vi "Start Transfer.vi"(8 "error in (no error)":errorcluster, 9 "finite?":bool=TRUE, 10 "stream index":i32, 11 "refnum in":refnum<k20>) -> (0 "error out":errorcluster, 3 "refnum out":refnum<k20>)   [LabVIEW 2015, in "niInstr Streaming v1 Host.lvlib"]
doc: "This low-level VI directly pokes the state machine to a started state (defined by the <b>finite?</b> paramter. This VI still waits for the state machine to report that it has left the idle state to ensure that the transfer has actually been started by the FPGA.\n\nThis VI provides no error checking. It does not check the state prior to execution, which may result in undesired behavior if the FPGA is in a bad state to start with. This VI should only be used by clients when they are asserting that the configuration and state are valid prior to calling this VI. However, because no error checking is performed, this VI may improve performance for starting a transfer.\n\n<B>Input Parameters</B>\n\n<B>error in (no error)</B> 'error in' can accept error information wired from VIs previously called. Use this information to decide if any functionality should be bypassed in the event of errors from other VIs.\n\nRight-click the 'error in' control on the front panel and select 'Explain Error' or 'Explain Warning' from the shortcut menu for more information about the error.\n\n<B>finite?</B> Indicates that this transfer should use the previously configured number of samples to transfer.\n\n<B>stream index</B> Selects which stream index this VI will interface to. This is the index number at the end of the host interface controls (0..7).\n\n<B>Output Parameters</B>\n\n<B>error out</B> contains error information. This output provides standard error out functionality.\n\n<B>refnum out</B> Copy of refnum in"
uses:
  <instrlib>/_niInstr/Streaming/v1/Host/niInstr Streaming v1 Host.lvlib
  <instrlib>/_niInstr/Streaming/v1/Common/Stream State.ctl
  <instrlib>/_niInstr/Streaming/v1/Common/niInstr Streaming v1 Common.lvlib
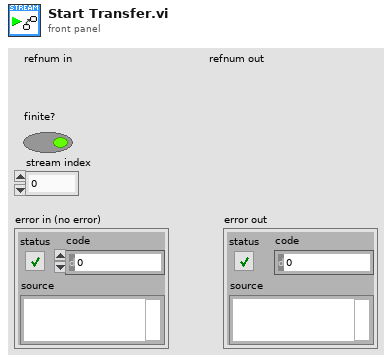
[diagram p1: front panel]
types:
  T1 = typedef "niInstr Streaming v1 Common.lvlib/Stream State.ctl" = enum8{"Idle", "Finite Transfer", "Continuous", "Done", "Error", "Not Ready", "Cancel"}
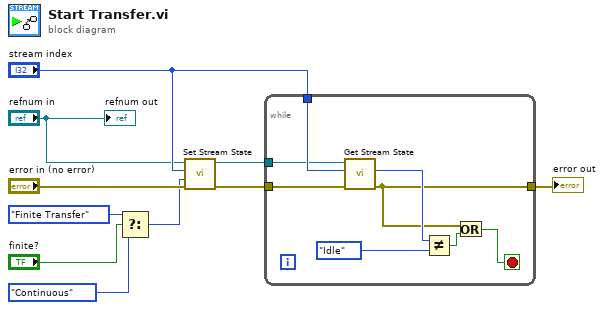
[diagram p0: block diagram]
diagram:
  n1 = Select(t=Stream_State."Finite Transfer" ("stream state"), s="finite?", f=Stream_State."Continuous" ("stream state")) -> (s? t:f=w2:T1)
  n2 = call <instrlib>:"Set Stream State.vi"("error in (no error)"="error in (no error)", "stream state"=w2, "stream index"="stream index", "refnum in"="refnum in") -> ("error out"=w7:errorcluster, "refnum out"=w8:refnum<k20>)  [unwired: 6 in]
  n3 = while {
    tunnel: "stream index" -> [w17]
    tunnel: w8 -> [w16]
    tunnel: w7 -> [w18]
    tunnel: [w11] -> w10
    stop <- w12 stop-if-true
    n4 = call <instrlib>:"Get Stream State.vi"("error in (no error)"=w18, "stream index"=w17, "refnum in"=w16) -> ("error out"=w11:errorcluster, "stream state"=w13:T1)  [unwired: 6 in, 1 out]
    n5 = Not Equal?(x=w13, y=Stream_State."Idle" ("stream.request state 0")) -> (x != y?=w15:bool)
    n6 = Or(x=w11, y=w15) -> (x .or. y?=w12:bool)
  }
  "error out" <- w10
  "refnum out" <- "refnum in"
